vi "Set Autorange.vi"(8 "error in (no error)":errorcluster, 11 "NI DMM Driver in":refnum<class "DMM.NI.lvclass">) -> (0 "error out":errorcluster, 3 "NI DMM Driver out":refnum<class "DMM.NI.lvclass">)   [LabVIEW 2020, in "NI DMM Driver.lvlib" / "DMM.NI.lvclass"]
doc: "Configure the DMM to autorange."
uses:
  DMM.NI.lvclass
  PPL/HDH.Driver.DMM.lvlibp/Controls/Ctl_DigitResolution.ctl
  PPL/HDH.Driver.DMM.lvlibp
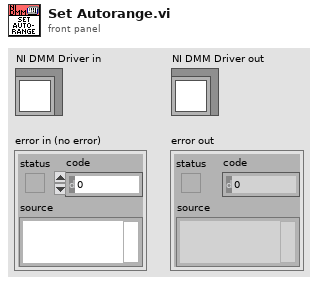
[diagram p1: front panel]
types:
  T1 = typedef "HDH.Driver.DMM.lvlibp/Ctl_DigitResolution.ctl" = enum8{"3½", "4½", "5½", "6½", "7½"}
  T2 = typedef "HDH.Driver.DMM.lvlibp/Ctl_Function.ctl" = enum8{"DC Volts", "AC Volts", "DC Current", "AC Current", "2-wire Resistance", "4-wire Resistance", "Diode", "Frequency", "Period", "AC Volts DC Coupled", "Capacitance", "Inductance", "Temperature"}
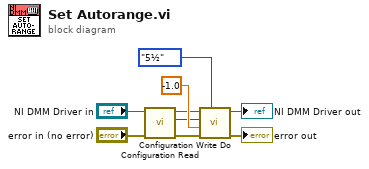
[diagram p0: block diagram]
diagram:
  n1 = call-dynamic "Configuration Read.vi"("error in (no error)"="error in (no error)", "NI DMM Driver in"="NI DMM Driver in") -> ("error out"=w2:errorcluster, "Function"=w5:T2, "NI DMM Driver out"=w4:refnum<class "DMM.NI.lvclass">)  [unwired: 5 in, 2 out]
  n2 = call-dynamic "Configuration Write Do.vi"("Digit Resolution(5½)"=Ctl_DigitResolution."5½", "error in (no error)"=w2, "Range"=-1.0, "Function"=w5, "NI DMM Driver in"=w4) -> ("error out"=→"error out":errorcluster, "NI DMM Driver out"=→"NI DMM Driver out":refnum<class "DMM.NI.lvclass">)  [unwired: 4 in, 1 out]
